vi "Write CVT.vi"(8 "error in (no error)":errorcluster, 10 "CVT":variant, 11 "CVT in":refnum<class "CVT.lvclass">) -> (0 "error out":errorcluster, 3 "CVT out":refnum<class "CVT.lvclass">)   [LabVIEW 2015, in "CVT.lvclass"]
uses:
  CVT.lvclass
  CVT.lvclass/CVT.ctl
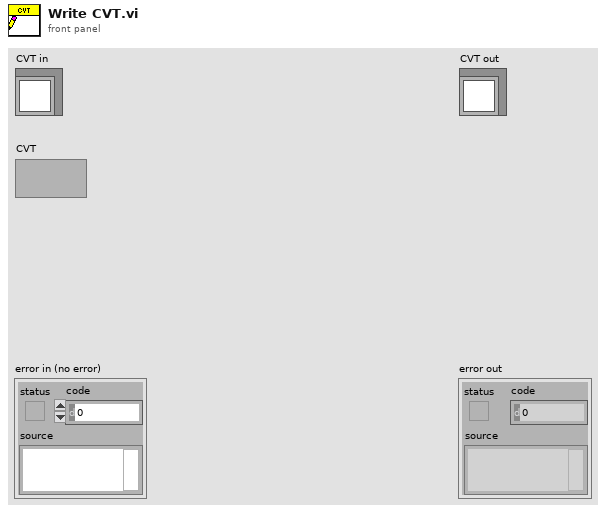
[diagram p1: front panel]
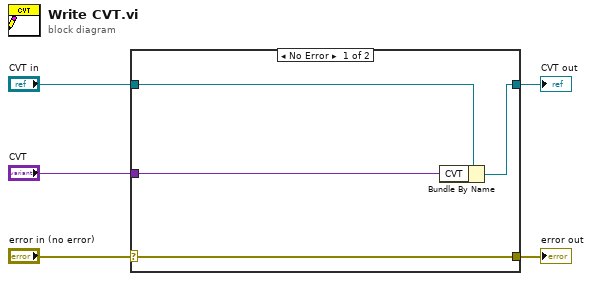
[diagram p0: block diagram]
diagram:
  n1 = case shown="No Error" "error in (no error)" {
    selector: "error in (no error)" -> [w9 w10]
    tunnel: [w9 w10] -> w4
    tunnel: [w7 w11] -> w2
    tunnel: "CVT in" -> [w8 w11]
    tunnel: "CVT" -> [w6 _]
    frame No Error {
      n2 = Bundle By Name(cluster=w8, "CVT"=w6) -> (w7:refnum<class "CVT.lvclass">)
    }
    frame Error {
    }
  }
  "error out" <- w4
  "CVT out" <- w2
